vi "MatrixReset.vi"(8 "error in (no error)":errorcluster, 11 "KE3700A in":refnum<class "KE3706A.lvclass">) -> (0 "error out":errorcluster, 3 "KE3700A out":refnum<class "KE3706A.lvclass">)   [LabVIEW 2013, in "KE3706A.lvclass"]
uses:
  KE3706A.lvclass
  Switching.lvclass
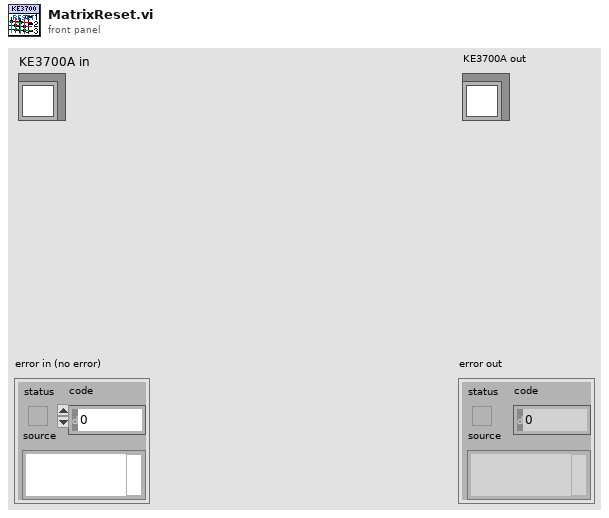
[diagram p1: front panel]
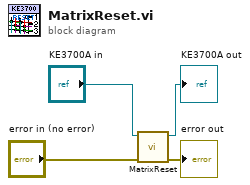
[diagram p0: block diagram]
diagram:
  n1 = call-parent "MatrixReset.vi"("error in (no error)"="error in (no error)", "Switching in"="KE3700A in") -> ("error out"=→"error out":errorcluster, "Switching out"=→"KE3700A out":refnum<class "KE3706A.lvclass">)  [unwired: 8 in]
